vi "Post Process Photon Counting.vi"(0 "pInputImage":i32, 1 "pOutputImage":i32, 2 "iOutputBufferSize":i32, 3 "iNumImages":i32, 4 "iNumframes":i32, 5 "iNumberOfThresholds":i32, 6 "pfThreshold":sgl, 7 "error in (no error)":errorcluster, 8 "iHeight":i32, 9 "iWidth":i32) -> (20 "pInputImage out":i32, 21 "pOutputImage out":i32, 22 "function return":u32, 26 "pfThreshold out":sgl, 27 "error out":errorcluster)   [LabVIEW 2014, in "atmcd32d.lvlib"]
doc: "unsigned int WINAPI PostProcessPhotonCounting(at_32 * pInputImage, at_32 * pOutputImage, int iOutputBufferSize, int iNumImages, int iNumframes, int iNumberOfThresholds, float * pfThreshold, int iHeight, int iWidth);"
uses:
  atmcd32d.lvlib
  atmcd32d.dll
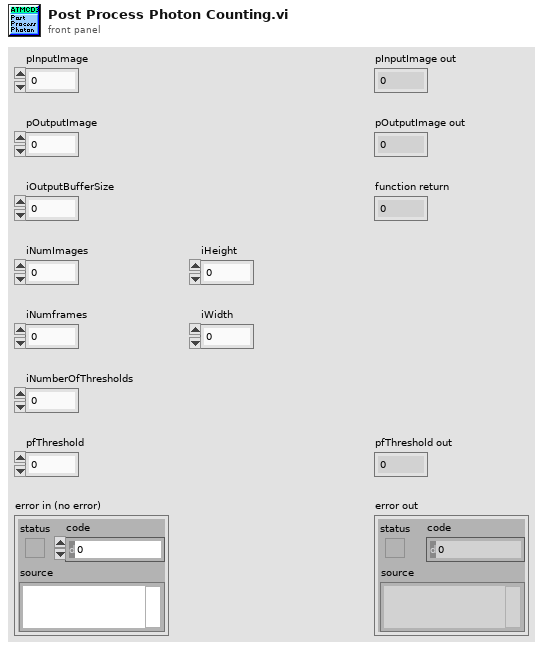
[diagram p1: front panel]
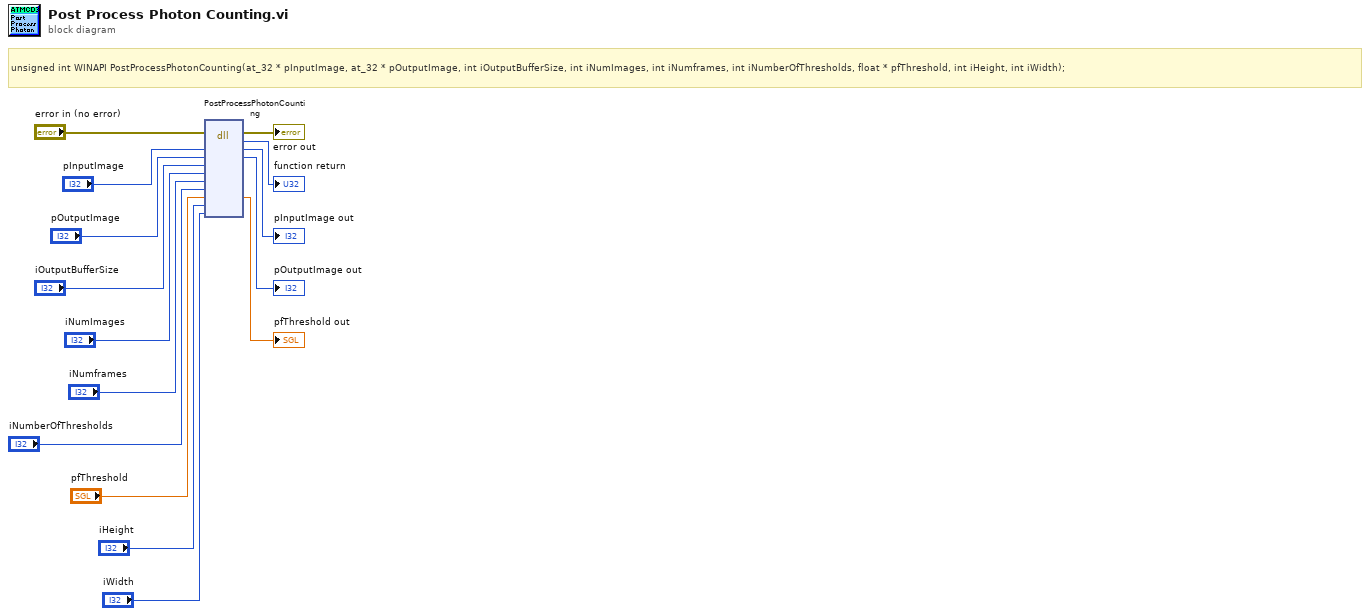
[diagram p0: block diagram]
diagram:
  # "unsigned int WINAPI PostProcessPhotonCounting(at_32 * pInputImage, at_32 * pOutputImage, int iOutputBufferSize, int iNumImages, int iNumframes, int iNumberOfThresholds, float * pfThreshold, int iHeight, int iWidth);"
  n1 = dll-call lib="C:/Users/Bakir/Documents/Lambda2-Testing/lib/Andorlib/atmcd32d.*" fn="PostProcessPhotonCounting"(error in="error in (no error)", "pInputImage"="pInputImage", "pOutputImage"="pOutputImage", "iOutputBufferSize"="iOutputBufferSize", "iNumImages"="iNumImages", "iNumframes"="iNumframes", "iNumberOfThresholds"="iNumberOfThresholds", "pfThreshold"="pfThreshold", "iHeight"="iHeight", "iWidth"="iWidth") -> (error out=→"error out":errorcluster, →"function return":u32, "pInputImage"=→"pInputImage out":i32, "pOutputImage"=→"pOutputImage out":i32, "pfThreshold"=→"pfThreshold out":sgl)  [unwired: 8 in, 1 out]
